vi "goto location.vi"(0 "Image Data":T2) -> (1 "left speed":dbl, 2 "right speed":dbl)   [LabVIEW 2013]
uses:
  typedefs/vision data.ctl
  typedefs/subStates.ctl
  <vilib>/addons/control/pid/pid.llb/PID (DBL).vi
  <vilib>/addons/control/pid/NI_PID_pid.lvlib
panel:
  in  "output range":cluster{"output high":dbl, "output low":dbl}={"output high"=0.5, "output low"=-0.5}
  in  "cutoff distance":dbl=0.25 format="%#_13g"
  in  "PID gains":T1={"proportional gain (Kc)"=1.0, "integral time (Ti, min)"=0.01, "derivative time (Td, min)"=0.0}
  # "Things needing Tuning"
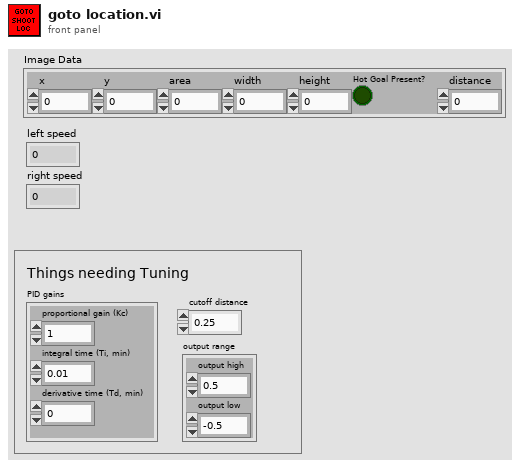
[diagram p1: front panel]
types:
  T1 = cluster{"proportional gain (Kc)":dbl, "integral time (Ti, min)":dbl, "derivative time (Td, min)":dbl}
  T2 = typedef "vision data.ctl" = cluster{"x":dbl, "y":dbl, "area":dbl, "width":dbl, "height":dbl, "Hot Goal Present?":bool, "distance":dbl}
  T3 = typedef "WPI_EncoderDevRef.ctl" = cluster{"DevStatus":errorcluster, "EncoderIndex":T4, "CounterIndex":T5, "DistancePerCount":dbl, "Decoding Type":T6}
  T4 = typedef "FPGA_EncoderIdx.ctl" = enum8{"Enc 0", "Enc 1", "Enc 2", "Enc 3", "Invalid"}
  T5 = typedef "FPGA_CounterCtrSystemIndex.ctl" = enum8{"Ctr 0", "Ctr 1", "Ctr 2", "Ctr 3", "Ctr 4", "Ctr 5", "Ctr 6", "Ctr 7", "Invalid"}
  T6 = typedef "WPI_EncoderType.ctl" = enum16{"1x", "2x", "4x"}
  T7 = cluster{"x":bool, "y":bool, "area":bool, "width":bool, "height":bool, "Hot Goal Present?":bool, "distance":bool}
  T8 = typedef "subStates.ctl" = enum16{"null", "wait", "driver control", "auto", "manual override", "hold position", "rotate", "pickup", "pass", "load", "goto shoot", "shoot", "end"}
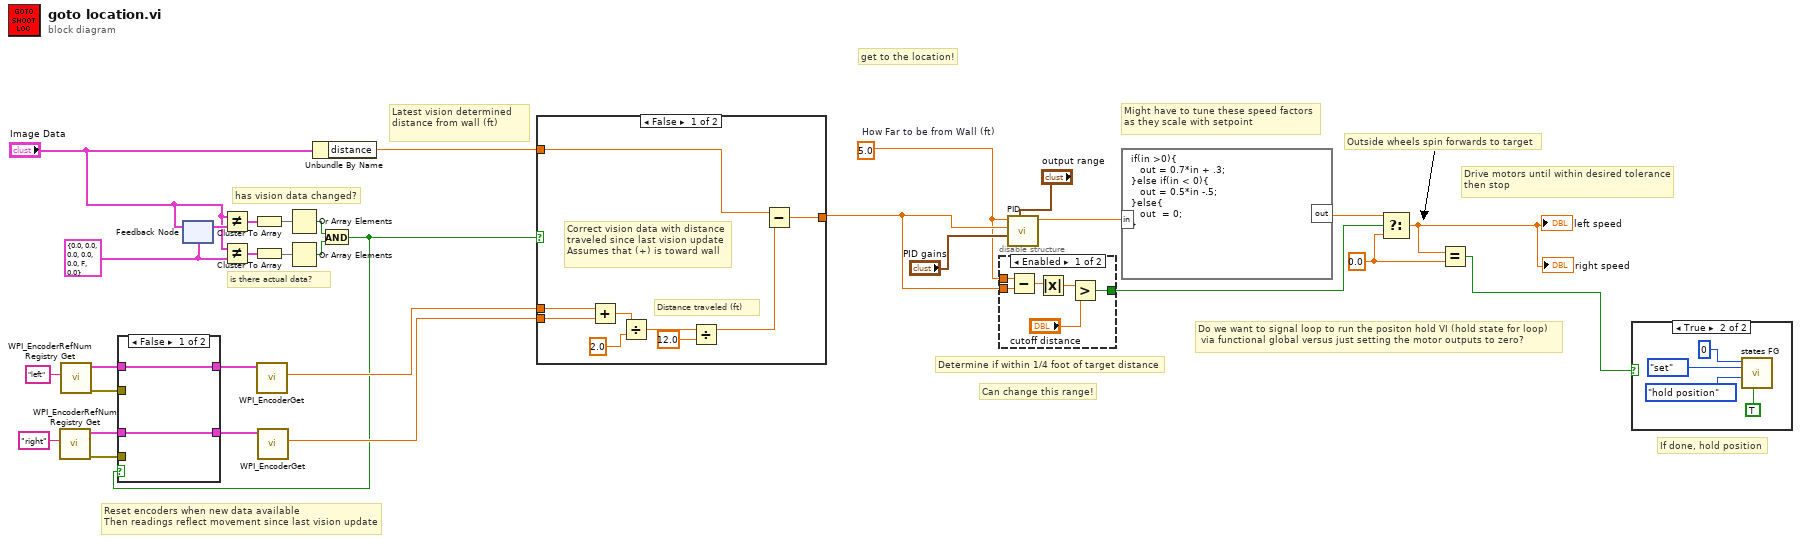
[diagram p0: block diagram]
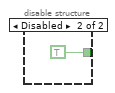
[diagram p3: hidden frame]
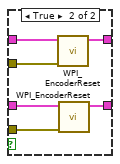
[diagram p5: hidden frame]
diagram:
  w5 = 5.0  # How Far to be from Wall (ft)
  w2 = 0.0 ("f")
  w23 = T2 {"x"=0.0, "y"=0.0, "area"=0.0, "width"=0.0, "height"=0.0, "Hot Goal Present?"=FALSE, "distance"=0.0} ("Image Data")
  # "If done, hold position"
  # "Might have to tune these speed factors\nas they scale with setpoint"
  # "Do we want to signal loop to run the positon hold VI (hold state for loop)\n via functional global versus just setting the motor outputs to zero?"
  # "Latest vision determined \ndistance from wall (ft)"
  # "Can change this range!"
  # "Determine if within 1/4 foot of target distance"
  # "Drive motors until within desired tolerance\nthen stop"
  # "get to the location!"
  # "Reset encoders when new data available\nThen readings reflect movement since last vision update"
  # "Outside wheels spin forwards to target"
  # "is there actual data?"
  # "has vision data changed?"
  n1 = call <vilib>:"WPI_EncoderRefNum Registry Get.vi"("refnum name"="right") -> ("error out"=w17:errorcluster, "EncoderDevRef"=w18:T3)  [unwired: 9 in]
  n2 = call <vilib>:"WPI_EncoderRefNum Registry Get.vi"("refnum name"="left") -> ("error out"=w19:errorcluster, "EncoderDevRef"=w20:T3)  [unwired: 9 in]
  n3 = feedback #1(w23) -> (w28:T2)
  n4 = feedback-in #1("Image Data") -> ()
  n5 = Not Equal?(x="Image Data", y=w28) -> (x != y?=w31:T7)
  n6 = Not Equal?(x="Image Data", y=w23) -> (x != y?=w29:T7)
  n7 = Cluster To Array(cluster=w31) -> (array=w30:bool[])
  n8 = Cluster To Array(cluster=w29) -> (array=w26:bool[])
  n9 = Or Array Elements(Boolean array=w30) -> (logical OR=w27:bool)
  n10 = Or Array Elements(Boolean array=w26) -> (logical OR=w25:bool)
  n11 = Unbundle By Name("Image Data") -> ("distance"=w4:dbl)
  n12 = And(x=w27, y=w25) -> (x .and. y?=w7:bool)
  n13 = case shown="False" w7 {
    tunnel: w20 -> [w33 w39]
    tunnel: w19 -> [_ w38]
    tunnel: w18 -> [w32 w37]
    tunnel: w17 -> [_ w36]
    tunnel: [w33 w35] -> w16
    tunnel: [w32 w34] -> w15
    frame False {
    }
    frame True {
      n14 = call <vilib>:"WPI_EncoderReset.vi"("error in (no error)"=w38, "EncoderDevRef"=w39) -> ("EncoderDevRef"=w35:T3)  [unwired: 8 in, 1 out]
      n15 = call <vilib>:"WPI_EncoderReset.vi"("error in (no error)"=w36, "EncoderDevRef"=w37) -> ("EncoderDevRef"=w34:T3)  [unwired: 8 in, 1 out]
    }
  }
  n16 = call <vilib>:"WPI_EncoderGet.vi"("EncoderDevRef"=w16) -> ("Distance"=w14:dbl)  [unwired: 5 in, 5 out]
  n17 = call <vilib>:"WPI_EncoderGet.vi"("EncoderDevRef"=w15) -> ("Distance"=w13:dbl)  [unwired: 5 in, 5 out]
  n18 = case shown="False" w7 {
    tunnel: w14 -> [w46 _]
    tunnel: w13 -> [w45 _]
    tunnel: w4 -> [w44 w49]
    tunnel: [w42 w49] -> w6
    frame False {
      # "Distance traveled (ft)"
      # "Correct vision data with distance \ntraveled since last vision update\nAssumes that (+) is toward wall"
      n19 = Add(x=w46, y=w45) -> (x+y=w47:dbl)
      n20 = Divide(x=w47, y=2.0) -> (x/y=w43:dbl)
      n21 = Divide(x=w43, y=12.0) -> (x/y=w41:dbl)
      n22 = Subtract(x=w44, y=w41) -> (x-y=w42:dbl)
    }
    frame True {
      # "Use visually determined distance"
    }
  }
  n23 = disable-structure shown="Enabled" {
    disable-tunnel: w6 -> [w54 _]
    disable-tunnel: [w51 TRUE] -> w8
    disable-tunnel: w5 -> [w50 _]
    frame Enabled {
      n24 = Subtract(x=w50, y=w54) -> (x-y=w55:dbl)
      n25 = Absolute Value(x=w55) -> (abs(x)=w53:dbl)
      n26 = Greater?(x=w53, y="cutoff distance") -> (0:w51:bool)
    }
    frame Disabled {
    }
  }
  n27 = call-poly <vilib>:"PID.vi"("output range"="output range", "PID gains"="PID gains", "process variable"=w6, "setpoint"=w5) -> ("output"=w11:dbl)  [unwired: 6 in, 1 out]
  n28 = formula code="if(in >0){\n   out = 0.7*in + .3;\n}else if(in < 0){\n   out = 0.5*in -.5;\n}else{\n   out  = 0;\n}"("in"=w11) -> ("out"=w12:dbl)
  n29 = Select(t=w12, s=w8, f=w2) -> (s? t:f=w3:dbl)
  "left speed" <- w3
  "right speed" <- w3
  n30 = Equal?(x=w3, y=w2) -> (x = y?=w1:bool)
  n31 = case shown="True" w1 {
    frame False {
    }
    frame True {
      n32 = call "states FG.vi"("exit in"=TRUE, "subState in"=subStates."hold position", "menu (get)"=enum16{"set", "get"}."set", "Loop ID"=0) -> ()  [unwired: 4 in, 4 out]
    }
  }
